vi "Intensity Graph.vi"() -> ()   [LabVIEW 2014]
panel:
  out "Waveform Graph":dbl[][](graph)
  out "Intensity Chart":dbl[][](graph)
  out "Intensity Graph":dbl[][](graph)
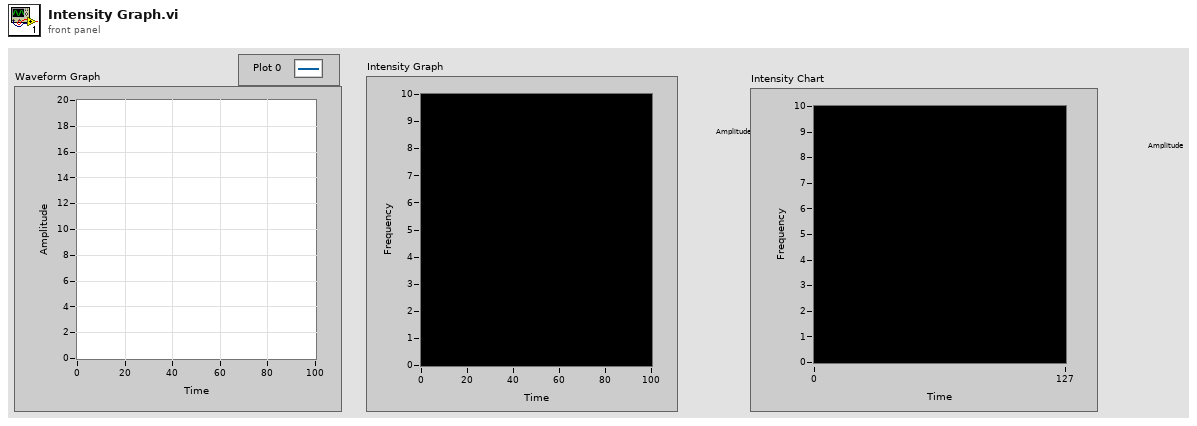
[diagram p1: front panel]
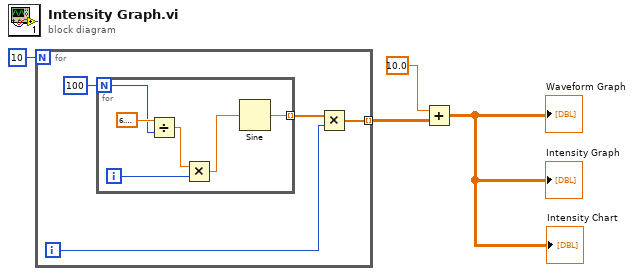
[diagram p0: block diagram]
diagram:
  n1 = for {
    N: 10 -> [_]
    tunnel: [w5] -> w3 mode=indexing
    i -> [w6]
    n2 = for {
      N: 100 -> [w13]
      tunnel: [w9] -> w7 mode=indexing
      i -> [w12]
      n3 = Divide(x=6.283185307179586, y=w13) -> (x/y=w11:dbl)
      n4 = Multiply(x=w11, y=w12) -> (x*y=w10:dbl)
      n5 = Sine(x=w10) -> (sin(x)=w9:dbl)
    }
    n6 = Multiply(x=w7, y=w6) -> (x*y=w5:dbl[])
  }
  n7 = Add(x=10.0, y=w3) -> (x+y=→"Intensity Graph" →"Intensity Chart" →"Waveform Graph":dbl[][])
